vi "find descriptor.vi"(1 "Circles":cluster{"x":dbl, "y":dbl, "r":dbl}[](array[cluster])) -> (0 "d":dbl[](array[numeric]))   [LabVIEW 2015]
panel:
  out "x":dbl[](array[numeric])
  out "y":dbl[](array[numeric])
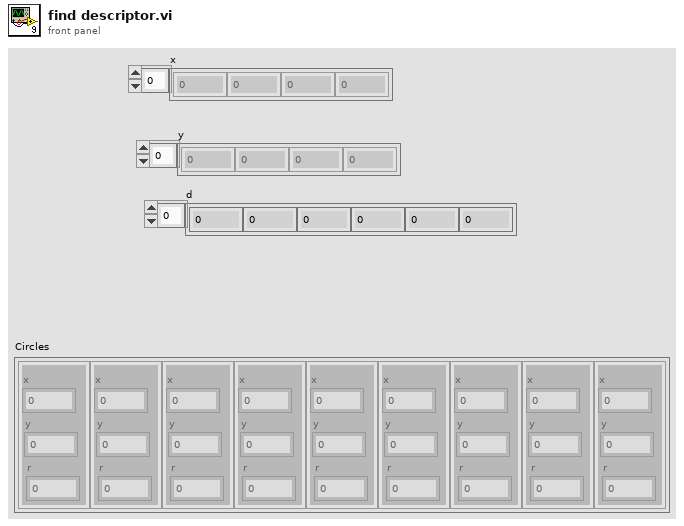
[diagram p1: front panel]
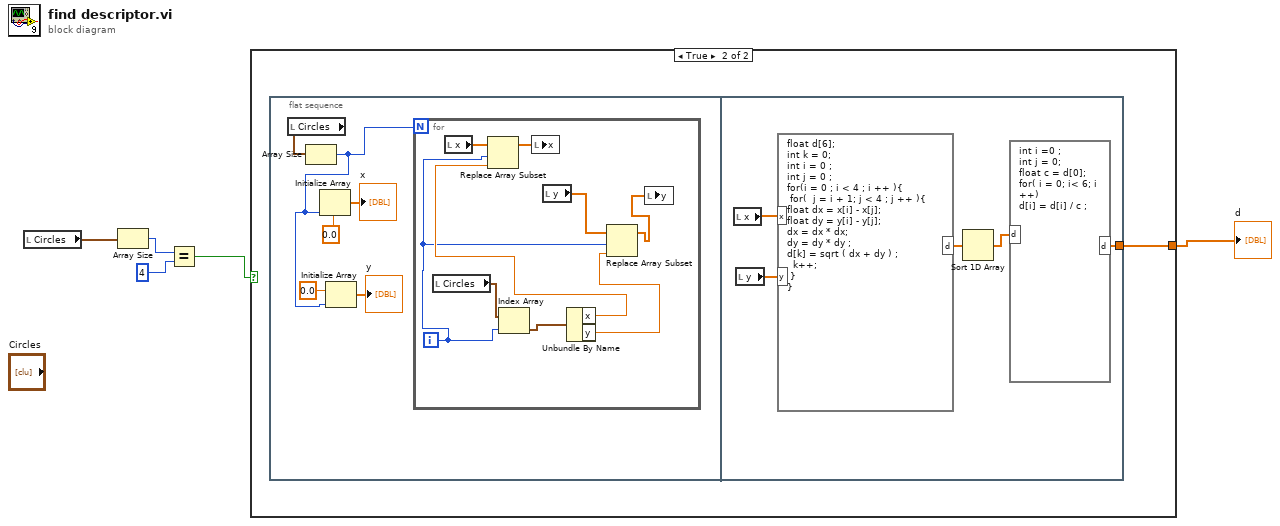
[diagram p0: block diagram]
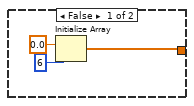
[diagram p2: hidden frame]
diagram:
  n1 = local read "Circles"() -> (w4:cluster{"x":dbl, "y":dbl, "r":dbl}[])
  n2 = Array Size(array=w4) -> (size(s)=w3:i32)
  n3 = Equal?(x=w3, y=4) -> (x = y?=w1:bool)
  n4 = case shown="True" w1 {
    tunnel: [w6 w9] -> w5
    frame False {
      n5 = Initialize Array(0.0 ("element"), 6 ("dimension size")) -> (w6:dbl[])
    }
    frame True {
      n6 = flat-sequence {
        tunnel: [w25] -> w9
        frame #0 {
          n7 = local read "Circles"() -> (w10:cluster{"x":dbl, "y":dbl, "r":dbl}[])
          n8 = Array Size(array=w10) -> (size(s)=w11:i32)
          n9 = Initialize Array(0.0 ("element"), w11) -> (→"x":dbl[])
          n10 = Initialize Array(0.0 ("element"), w11) -> (→"y":dbl[])
          n11 = for {
            N: w11 -> [_]
            i -> [w18]
            n12 = local read "Circles"() -> (w24:cluster{"x":dbl, "y":dbl, "r":dbl}[])
            n13 = local read "x"() -> (w22:dbl[])
            n14 = Index Array(array=w24, index=w18) -> (element=w23:cluster{"x":dbl, "y":dbl, "r":dbl})
            n15 = local read "y"() -> (w19:dbl[])
            n16 = Unbundle By Name(w23) -> ("x"=w21:dbl, "y"=w17:dbl)
            n17 = Replace Array Subset(array=w22, new element=w21, index=w18) -> (w20:dbl[])
            n18 = local write "x"(w20) -> ()
            n19 = Replace Array Subset(array=w19, new element=w17, index=w18) -> (w16:dbl[])
            n20 = local write "y"(w16) -> ()
          }
        }
        frame #1 {
          n21 = local read "x"() -> (w29:dbl[])
          n22 = local read "y"() -> (w28:dbl[])
          n23 = formula code="float d[6];\nint k = 0;\nint i = 0 ;\nint j = 0 ;\nfor(i = 0 ; i < 4 ; i ++ ){\n\tfor(  j = i + 1; j < 4 ; j ++ ){\nfloat dx = x[i] - x[j];\nfloat dy = y[i] - y[j];\ndx = dx * dx; \ndy = dy * dy ;\nd[k] = sqrt ( dx + dy ) ;\n\t\tk++;\n\t}\n}"("x"=w29, "y"=w28) -> ("d"=w27:dbl[])
          n24 = Sort 1D Array(array=w27) -> (sorted array=w26:dbl[])
          n25 = formula code="int i =0 ;\nint j = 0;\nfloat c = d[0];\nfor( i = 0; i< 6; i ++)\nd[i] = d[i] / c ;"("d"=w26) -> ("d"=w25:dbl[])
        }
      }
    }
  }
  "d" <- w5
